vi "Write Parent Data.vi"(8 "error in (no error)":errorcluster, 10 "Parent Data":dbl, 11 "Parent in":refnum<class "Parent.lvclass">) -> (0 "error out":errorcluster, 3 "Parent out":refnum<class "Parent.lvclass">)   [LabVIEW 2020, in "TEST - JKI JSON Object Serialization.lvlib" / "Parent.lvclass"]
uses:
  Parent.lvclass
  Parent.lvclass/Parent.ctl
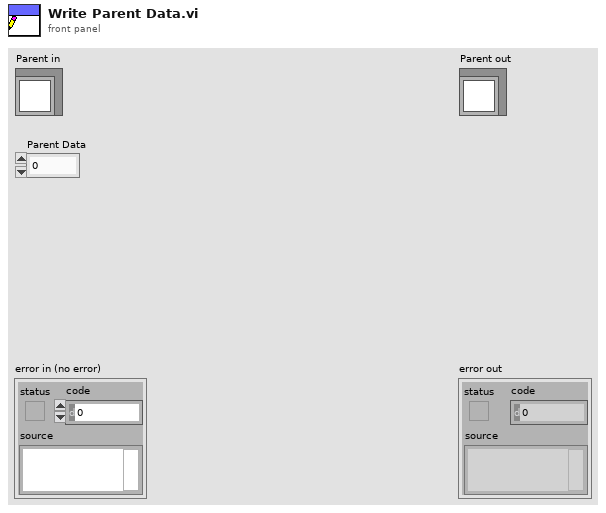
[diagram p1: front panel]
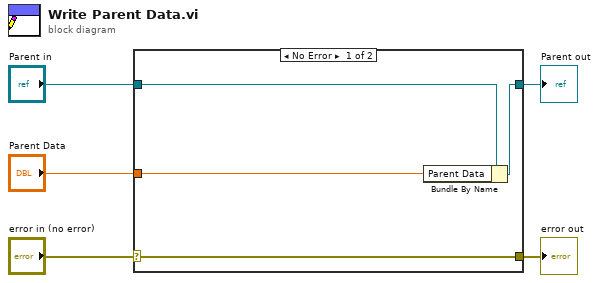
[diagram p0: block diagram]
diagram:
  n1 = case shown="No Error" "error in (no error)" {
    selector: "error in (no error)" -> [w9 w10]
    tunnel: [w9 w10] -> w4
    tunnel: [w7 w11] -> w2
    tunnel: "Parent in" -> [w8 w11]
    tunnel: "Parent Data" -> [w6 _]
    frame No Error {
      n2 = Bundle By Name(cluster=w8, "Parent Data"=w6) -> (w7:refnum<class "Parent.lvclass">)
    }
    frame Error {
    }
  }
  "error out" <- w4
  "Parent out" <- w2
